vi "Double Acquire Every Image (Optimized Performance).vi"() -> ()   [LabVIEW 2020]
doc: "The Acquire Every Image (Optimized Performance) example shows the basics of using a ring acquisition. There are some camera restrictions to using this mode that are described in more detail in the block diagram of the VI, but it is recommended to use this method for performance-critical applications when possible."
uses:
  <vilib>/vision/driver/IMAQdx.llb/IMAQdx Acquisition Mode.ctl
  <vilib>/vision/driver/IMAQdx.llb/IMAQdx Buffer Number Mode.ctl
  <vilib>/vision/driver/NI_Vision_Acquisition_Software.lvlib
  <resource>/objmgr/imaqdx.rc
panel:
  in  "Overwrite Mode 2":u16(ring) items=["Get Oldest"=0, "Fail"=2, "Get Newest"=3]
  in  "Number of Images 2":i32=10
  in  "Camera Name 2":refnum<k21> caption="IMAQdx Session"
  in  "Stop 2":bool
  out "Acquired Frame Rate 2":dbl
  out "Buffer Number 2":u32
  out "Images Behind 2":i32
  out "Processing Frame Rate 2":dbl
  out "Images Missed 2":u32
  out "Image 2":T1(plugin-control)
  in  "Simulated Processing Delay (ms) 2":i32
  in  "Overwrite Mode":u16(ring) items=["Get Oldest"=0, "Fail"=2, "Get Newest"=3]
  in  "Simulated Processing Delay (ms)":i32
  out "Images Missed":u32
  out "Images Behind":i32
  out "Processing Frame Rate":dbl
  in  "Number of Images":i32=10
  in  "Camera Name":refnum<k21> caption="IMAQdx Session"
  out "Buffer Number":u32
  out "Image":T1(plugin-control)
  out "Acquired Frame Rate":dbl
  in  "Stop":bool
  # "Overview: Demonstrates how to acquire continuous images using a ring acquisition, which is optimized for performance.\nRequirements: Vision Acquisition Software\nInstructions:\n1. Select the Camera Name\n2. Run the VI\n3. Increase the Simulated Processing Delay to see the effect on Images Behind and Images Missed when the acquisition loop isn't executed as quickly as the camera acquires images."
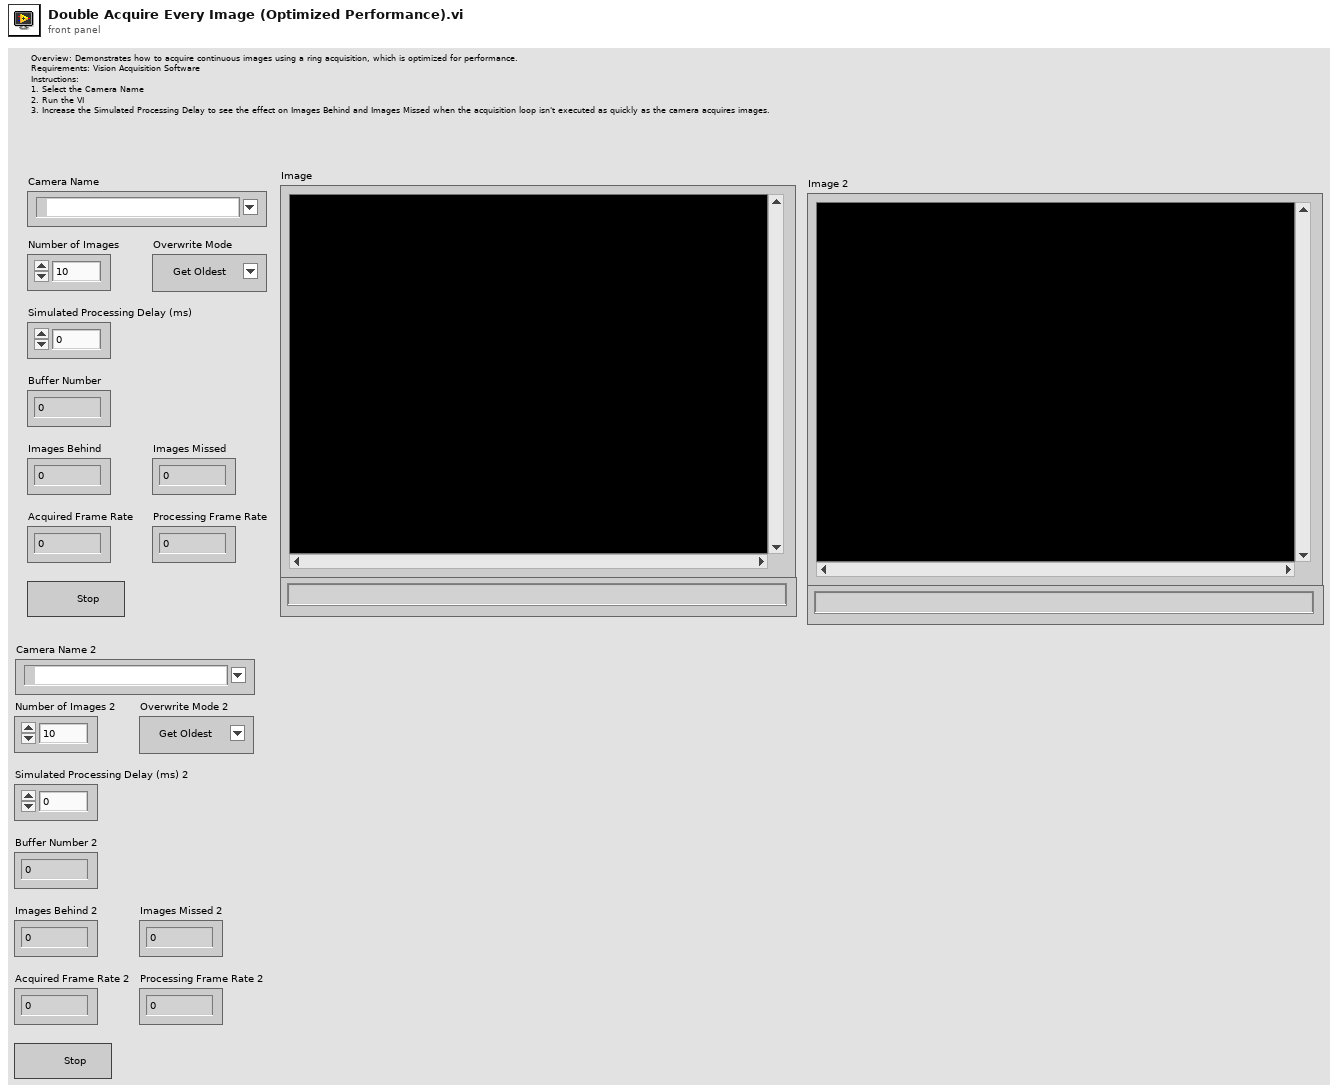
[diagram p1: front panel]
types:
  T1 = typedef "IMAQ Image.ctl" = refnum<image>
  T2 = typedef "NI_Vision_Acquisition_Software.lvlib/IMAQdx Acquisition Mode.ctl" = enum32{"One Shot", "Continuous"}
  T3 = typedef "IMAQdx.ctl" = refnum<k21>
  T4 = typedef "NI_Vision_Acquisition_Software.lvlib/IMAQdx Buffer Number Mode.ctl" = enum32{"Next", "Last", "Buffer Number", "Every", "Last New"}
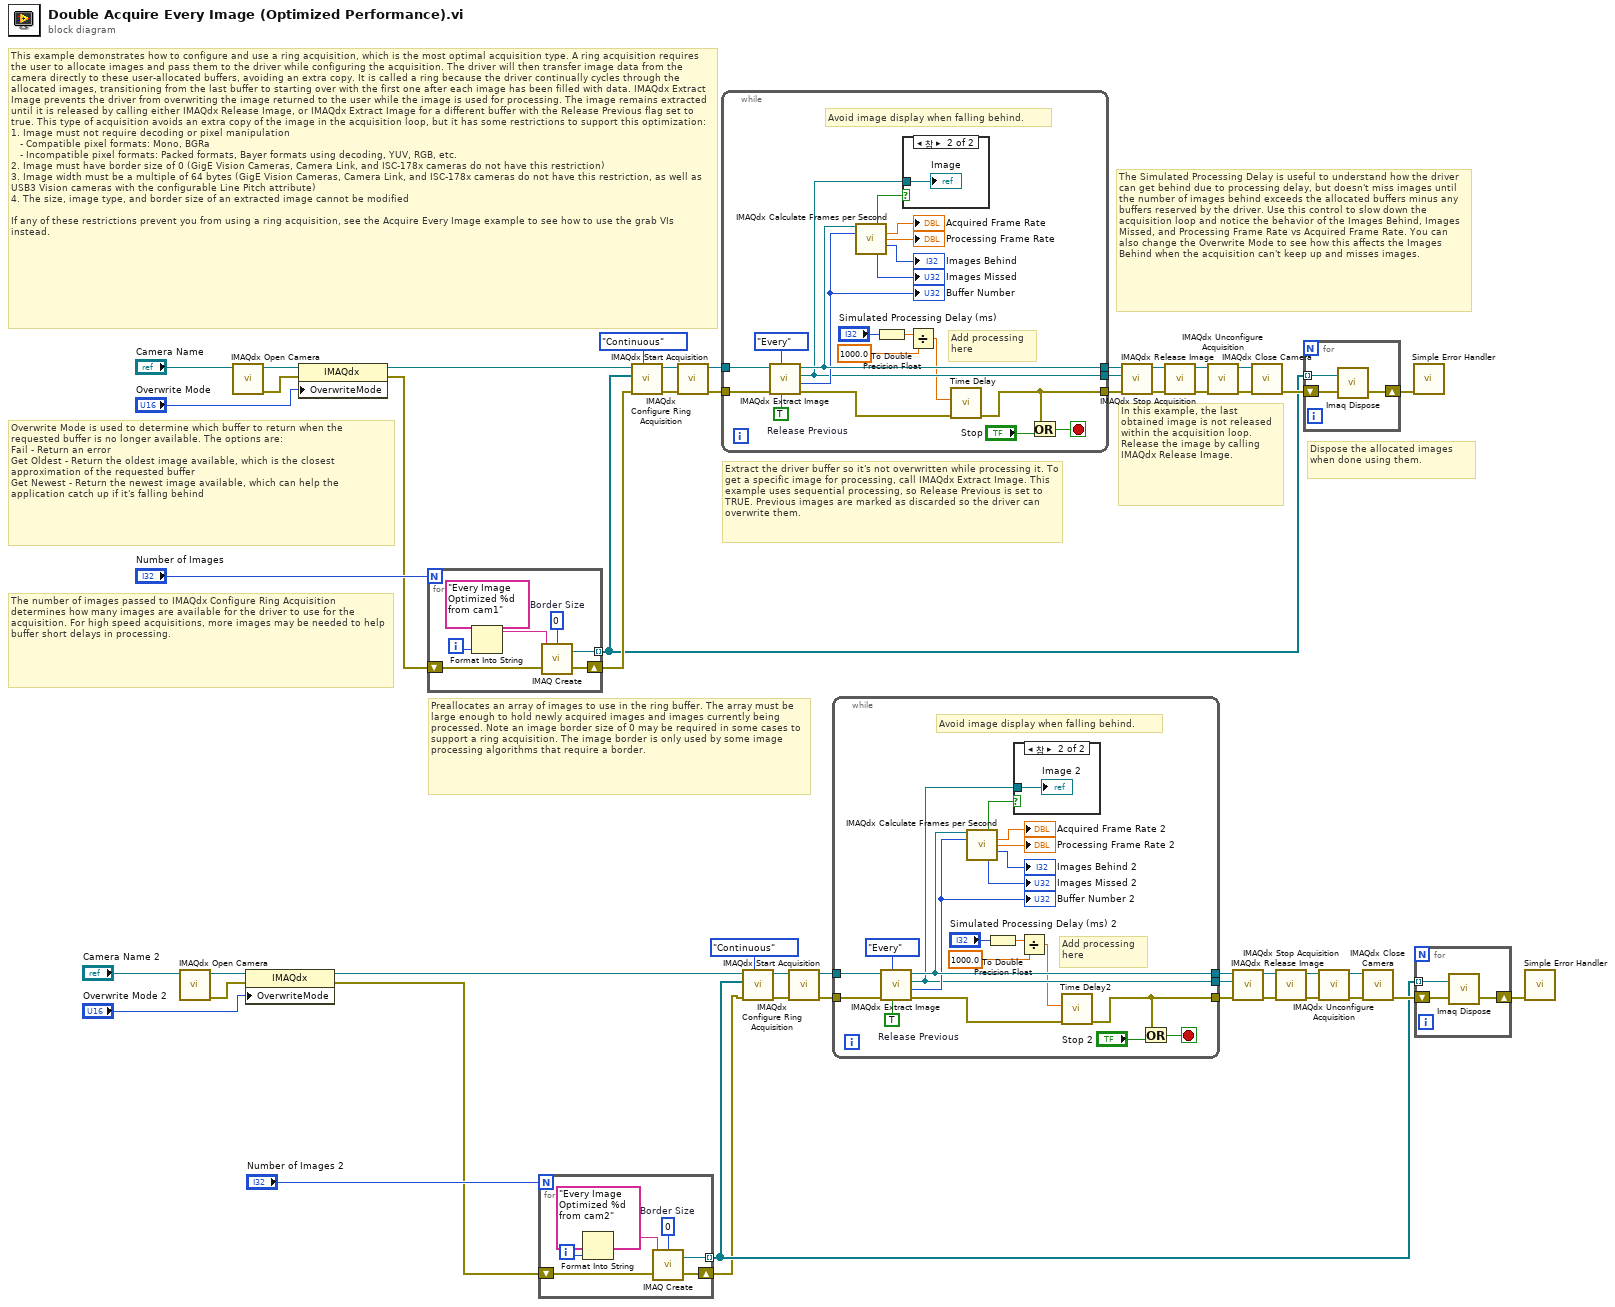
[diagram p0: block diagram]
diagram:
  # "The Simulated Processing Delay is useful to understand how the driver can get behind due to processing delay, but doesn't miss images until the number of images behind exceeds the allocated buffers minus any buffers reserved by the driver. Use this control to slow down the acquisition loop and notice the behavior of the Images Behind, Images Missed, and Processing Frame Rate vs Acquired Frame Rate. You can also change the Overwrite Mode to see how this affects the Images Behind when the acquisition can't keep up and misses images."
  # "Dispose the allocated images when done using them."
  # "The number of images passed to IMAQdx Configure Ring Acquisition determines how many images are available for the driver to use for the acquisition. For high speed acquisitions, more images may be needed to help buffer short delays in processing."
  # "Overwrite Mode is used to determine which buffer to return when the requested buffer is no longer available. The options are:\nFail - Return an error\nGet Oldest - Return the oldest image available, which is the closest approximation of the requested buffer\nGet Newest - Return the newest image available, which can help the application catch up if it's falling behind"
  # "This example demonstrates how to configure and use a ring acquisition, which is the most optimal acquisition type. A ring acquisition requires the user to allocate images and pass them to the driver while configuring the acquisition. The driver will then transfer image data from the camera directly to these user-allocated buffers, avoiding an extra copy. It is called a ring because the driver continually cycles through the allocated images, transitioning from the last buffer to starting over with the first one after each image has been filled with data. IMAQdx Extract Image prevents the driver from overwriting the image returned to the user while the image is used for processing. The image remains extracted until it is released by calling either IMAQdx Release Image, or IMAQdx Extract Image for a different buffer with the Release Previous flag set to true. This type of acquisition avoids an extra copy of the image in the acquisition loop, but it has some restrictions to support this optimization:\n1. Image must not require decoding or pixel manipulation\n   - Compatible pixel formats: Mono, BGRa\n   - Incompatible pixel formats: Packed formats, Bayer formats using decoding, YUV, RGB, etc.\n2. Image must have border size of 0 (GigE Vision Cameras, Camera Link, and ISC-178x cameras do not have this restriction)\n3. Image width must be a multiple of 64 bytes (GigE Vision Cameras, Camera Link, and ISC-178x cameras do not have this restriction, as well as USB3 Vision cameras with the configurable Line Pitch attribute)\n4. The size, image type, and border size of an extracted image cannot be modified\n\nIf any of these restrictions prevent you from using a ring acquisition, see the Acquire Every Image example to see how to use the grab VIs instead."
  # "In this example, the last obtained image is not released within the acquisition loop. Release the image by calling IMAQdx Release Image."
  # "Extract the driver buffer so it's not overwritten while processing it. To get a specific image for processing, call IMAQdx Extract Image. This example uses sequential processing, so Release Previous is set to TRUE. Previous images are marked as discarded so the driver can overwrite them."
  # "Preallocates an array of images to use in the ring buffer. The array must be large enough to hold newly acquired images and images currently being processed. Note an image border size of 0 may be required in some cases to support a ring acquisition. The image border is only used by some image processing algorithms that require a border."
  n1 = call <vilib>:"IMAQdx Open Camera.vi"("Session In"="Camera Name 2") -> ("error out"=w4:errorcluster, "Session Out"=w6:T3)  [unwired: 2 in, 7 out]
  n2 = call <vilib>:"IMAQdx Open Camera.vi"("Session In"="Camera Name") -> ("error out"=w28:errorcluster, "Session Out"=w30:T3)  [unwired: 2 in, 7 out]
  n3 = property class="IMAQdx"(reference=w6, error in=w4, "OverwriteMode"="Overwrite Mode 2") -> (reference out=w5:T3, error out=w2:errorcluster)
  n4 = property class="IMAQdx"(reference=w30, error in=w28, "OverwriteMode"="Overwrite Mode") -> (reference out=w29:T3, error out=w27:errorcluster)
  n5 = for {
    N: "Number of Images" -> [_]
    tunnel: [w56] -> w31 mode=indexing
    shift-right: [w55] -> w38
    shift-left: w27 -> [w57]
    i -> [w54]
    w51 = 0  # Border Size
    n6 = Format Into String(format string="Every Image Optimized %d from cam1" ("Image Name"), w54) -> (resulting string=w53:string)  [unwired: 2 in, 1 out]
    n7 = call "IMAQ Create"("Border Size"=w51, "Image Name"=w53, "error in (no error)"=w57) -> ("New Image"=w56:T1, "error out"=w55:errorcluster)  [unwired: 1 in, 1 out]
  }
  n8 = for {
    N: "Number of Images 2" -> [_]
    tunnel: [w64] -> w7 mode=indexing
    shift-right: [w58] -> w1
    shift-left: w2 -> [w59]
    i -> [w63]
    w60 = 0  # Border Size
    n9 = Format Into String(format string="Every Image Optimized %d from cam2" ("Image Name"), w63) -> (resulting string=w62:string)  [unwired: 2 in, 1 out]
    n10 = call "IMAQ Create"("Border Size"=w60, "Image Name"=w62, "error in (no error)"=w59) -> ("New Image"=w64:T1, "error out"=w58:errorcluster)  [unwired: 1 in, 1 out]
  }
  n11 = call <vilib>:"IMAQdx Configure Ring Acquisition.vi"("Mode"=IMAQdx_Acquisition_Mode."Continuous" ("Continuous?"), "error in"=w38, "Images"=w31, "Session In"=w29) -> ("error out"=w39:errorcluster, "Session Out"=w40:T3)  [unwired: 5 in, 1 out]
  n12 = call <vilib>:"IMAQdx Start Acquisition.vi"("error in"=w39, "Session In"=w40) -> ("error out"=w48:errorcluster, "Session Out"=w49:T3)  [unwired: 8 out]
  n13 = while {
    tunnel: [w78] -> w33
    tunnel: w48 -> [w82]
    tunnel: w49 -> [w83]
    tunnel: [w72] -> w35
    tunnel: [w74] -> w36
    stop <- w84 stop-if-true
    w79 = TRUE  # Release Previous
    # "Avoid image display when falling behind."
    # "Add processing here"
    n14 = call <vilib>:"IMAQdx Extract Image.vi"("Release Previous (true)"=w79, "Buffer Number Mode (Next)"=IMAQdx_Buffer_Number_Mode."Every" ("Buffer Number Mode"), "error in"=w82, "Session In"=w83) -> ("error out"=w73:errorcluster, "Buffer Number Out"=w77:u32, "Image Out"=w74:T1, "Session Out"=w78:T3)  [unwired: 4 in]
    "Buffer Number" <- w77
    n15 = call <vilib>:"IMAQdx Calculate Frames per Second.vi"("Session In"=w78, "Buffer Number"=w77) -> ("Update Display"=w75:bool, "Acquired Frames per Second"=→"Acquired Frame Rate":dbl, "Processed Frames per Second"=→"Processing Frame Rate":dbl, "Images Behind"=→"Images Behind":i32, "Images Missed"=→"Images Missed":u32)  [unwired: 7 in, 2 out]
    n16 = To Double Precision Float(number="Simulated Processing Delay (ms)") -> (double precision float=w65:dbl)
    n17 = case shown="참" w75 {
      tunnel: w74 -> [_ w85]
      frame False {
      }
      frame True {
        "Image" <- w85
      }
    }
    n18 = Divide(x=w65, y=1000.0) -> (x/y=w69:dbl)
    n19 = call "Time Delay"("error in (no error)"=w73, "Delay Time (s)"=w69) -> ("error out"=w72:errorcluster)  [unwired: 9 in]
    n20 = Or(x=w72, y="Stop") -> (x .or. y?=w84:bool)
  }
  n21 = call <vilib>:"IMAQdx Configure Ring Acquisition.vi"("Mode"=IMAQdx_Acquisition_Mode."Continuous" ("Continuous?"), "error in"=w1, "Images"=w7, "Session In"=w5) -> ("error out"=w14:errorcluster, "Session Out"=w15:T3)  [unwired: 5 in, 1 out]
  n22 = call <vilib>:"IMAQdx Start Acquisition.vi"("error in"=w14, "Session In"=w15) -> ("error out"=w23:errorcluster, "Session Out"=w24:T3)  [unwired: 8 out]
  n23 = while {
    tunnel: [w99] -> w9
    tunnel: w23 -> [w103]
    tunnel: w24 -> [w104]
    tunnel: [w93] -> w11
    tunnel: [w95] -> w12
    stop <- w105 stop-if-true
    w100 = TRUE  # Release Previous
    # "Avoid image display when falling behind."
    # "Add processing here"
    n24 = call <vilib>:"IMAQdx Extract Image.vi"("Release Previous (true)"=w100, "Buffer Number Mode (Next)"=IMAQdx_Buffer_Number_Mode."Every" ("Buffer Number Mode"), "error in"=w103, "Session In"=w104) -> ("error out"=w94:errorcluster, "Buffer Number Out"=w98:u32, "Image Out"=w95:T1, "Session Out"=w99:T3)  [unwired: 4 in]
    "Buffer Number 2" <- w98
    n25 = call <vilib>:"IMAQdx Calculate Frames per Second.vi"("Session In"=w99, "Buffer Number"=w98) -> ("Update Display"=w96:bool, "Acquired Frames per Second"=→"Acquired Frame Rate 2":dbl, "Processed Frames per Second"=→"Processing Frame Rate 2":dbl, "Images Behind"=→"Images Behind 2":i32, "Images Missed"=→"Images Missed 2":u32)  [unwired: 7 in, 2 out]
    n26 = To Double Precision Float(number="Simulated Processing Delay (ms) 2") -> (double precision float=w86:dbl)
    n27 = case shown="참" w96 {
      tunnel: w95 -> [_ w106]
      frame False {
      }
      frame True {
        "Image 2" <- w106
      }
    }
    n28 = Divide(x=w86, y=1000.0) -> (x/y=w90:dbl)
    n29 = call "Time Delay2"("error in (no error)"=w94, "Delay Time (s)"=w90) -> ("error out"=w93:errorcluster)  [unwired: 9 in]
    n30 = Or(x=w93, y="Stop 2") -> (x .or. y?=w105:bool)
  }
  n31 = call <vilib>:"IMAQdx Release Image.vi"("error in"=w35, "Image"=w36, "Session In"=w33) -> ("error out"=w34:errorcluster, "Session Out"=w32:T3)  [unwired: 7 in]
  n32 = call <vilib>:"IMAQdx Stop Acquisition.vi"("error in"=w34, "Session In"=w32) -> ("error out"=w44:errorcluster, "Session Out"=w45:T3)  [unwired: 8 out]
  n33 = call <vilib>:"IMAQdx Unconfigure Acquisition.vi"("error in"=w44, "Session In"=w45) -> ("error out"=w47:errorcluster, "Session Out"=w46:T3)  [unwired: 8 out]
  n34 = call <vilib>:"IMAQdx Release Image.vi"("error in"=w11, "Image"=w12, "Session In"=w9) -> ("error out"=w10:errorcluster, "Session Out"=w8:T3)  [unwired: 7 in]
  n35 = call <vilib>:"IMAQdx Close Camera.vi"("error in"=w47, "Session In"=w46) -> ("error out"=w43:errorcluster)  [unwired: 9 out]
  n36 = call <vilib>:"IMAQdx Stop Acquisition.vi"("error in"=w10, "Session In"=w8) -> ("error out"=w19:errorcluster, "Session Out"=w20:T3)  [unwired: 8 out]
  n37 = for {
    shift-right: [w108] -> w42
    shift-left: w43 -> [w109]
    tunnel: w31 -> [w107] mode=indexing
    n38 = call "Imaq Dispose"("Image"=w107, "error in (no error)"=w109) -> ("error out"=w108:errorcluster)  [unwired: 4 in]
  }
  n39 = call <vilib>:"IMAQdx Unconfigure Acquisition.vi"("error in"=w19, "Session In"=w20) -> ("error out"=w22:errorcluster, "Session Out"=w21:T3)  [unwired: 8 out]
  n40 = call <vilib>:"IMAQdx Close Camera.vi"("error in"=w22, "Session In"=w21) -> ("error out"=w18:errorcluster)  [unwired: 9 out]
  n41 = call <vilib>:"Simple Error Handler.vi"("error in (no error)"=w42) -> ()  [unwired: 4 in, 5 out]
  n42 = for {
    shift-right: [w111] -> w17
    shift-left: w18 -> [w112]
    tunnel: w7 -> [w110] mode=indexing
    n43 = call "Imaq Dispose"("Image"=w110, "error in (no error)"=w112) -> ("error out"=w111:errorcluster)  [unwired: 4 in]
  }
  n44 = call <vilib>:"Simple Error Handler.vi"("error in (no error)"=w17) -> ()  [unwired: 4 in, 5 out]
